vi "createViPath.vi"(6 "CommandType":T1, 8 "error in (no error)":errorcluster, 9 "topic":string, 11 "ProgrammaticInitialization in":refnum<class "ProgrammaticInitialization.lvclass">) -> (0 "error out":errorcluster, 1 "vi name":string, 2 "path":path, 3 "ProgrammaticInitialization out":refnum<class "ProgrammaticInitialization.lvclass">)   [LabVIEW 2016, in "ProgrammaticInitialization.lvclass"]
uses:
  ProgrammaticInitialization.lvclass
  commandType.ctl
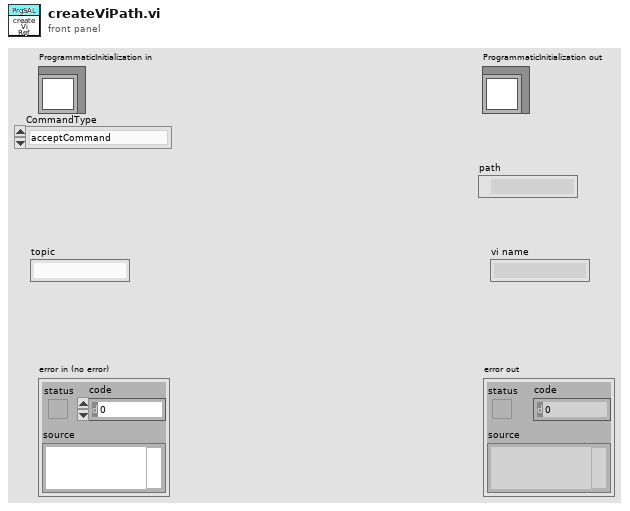
[diagram p1: front panel]
types:
  T1 = typedef "ProgrammaticInitialization.lvclass/commandType.ctl" = enum16{"acceptCommand", "ackCommand", "cancelCallback_command", "cancelCallback_logEvent", "cancelCallback", "flushSamplesEvent", "getEvent", "getNextSample", "getResponse", "getSample", "issueCommand", "logEvent", "monitorCommand", "putSample", "registerCallback_command", "registerCallback_logEvent", "registerCallback", "salCommander", "salEvent", "salProcessor", "salTelemetrySub", "waitForCompletion"}
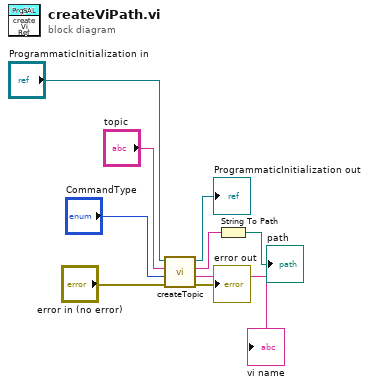
[diagram p0: block diagram]
diagram:
  n1 = call "createTopic.vi"("error in (no error)"="error in (no error)", "CommandType"="CommandType", "topic"="topic", "ProgrammaticInitialization in"="ProgrammaticInitialization in") -> ("error out"=→"error out":errorcluster, "vi name"=→"vi name":string, "topicVI"=w3:string, "ProgrammaticInitialization out"=→"ProgrammaticInitialization out":refnum<class "ProgrammaticInitialization.lvclass">)  [unwired: 4 in]
  n2 = String To Path(string=w3) -> (path=→"path":path)
